vi "8_2.vi"() -> ()   [LabVIEW 2021, in "2023.lvlib"]
uses:
  2023.lvlib
panel:
  out "x*y":i64
  out "product":i64
  out "lines":string[](array[string])
  in  "Demo / Real Input":bool
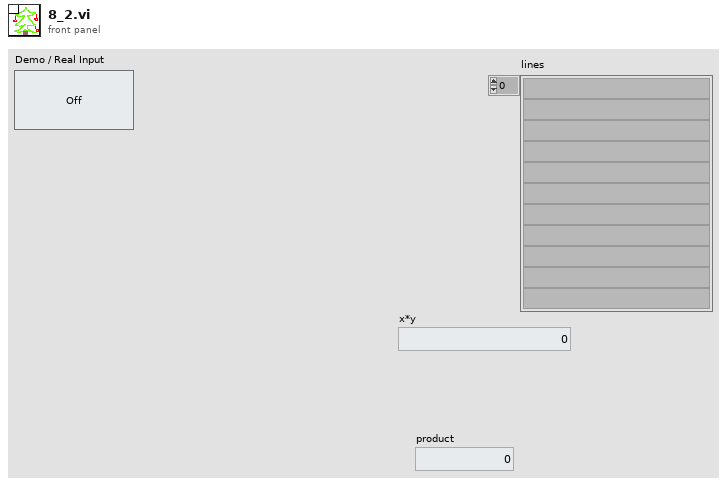
[diagram p1: front panel]
types:
  T1 = map{string, cluster{"LEFT":string, "RIGHT":string}}
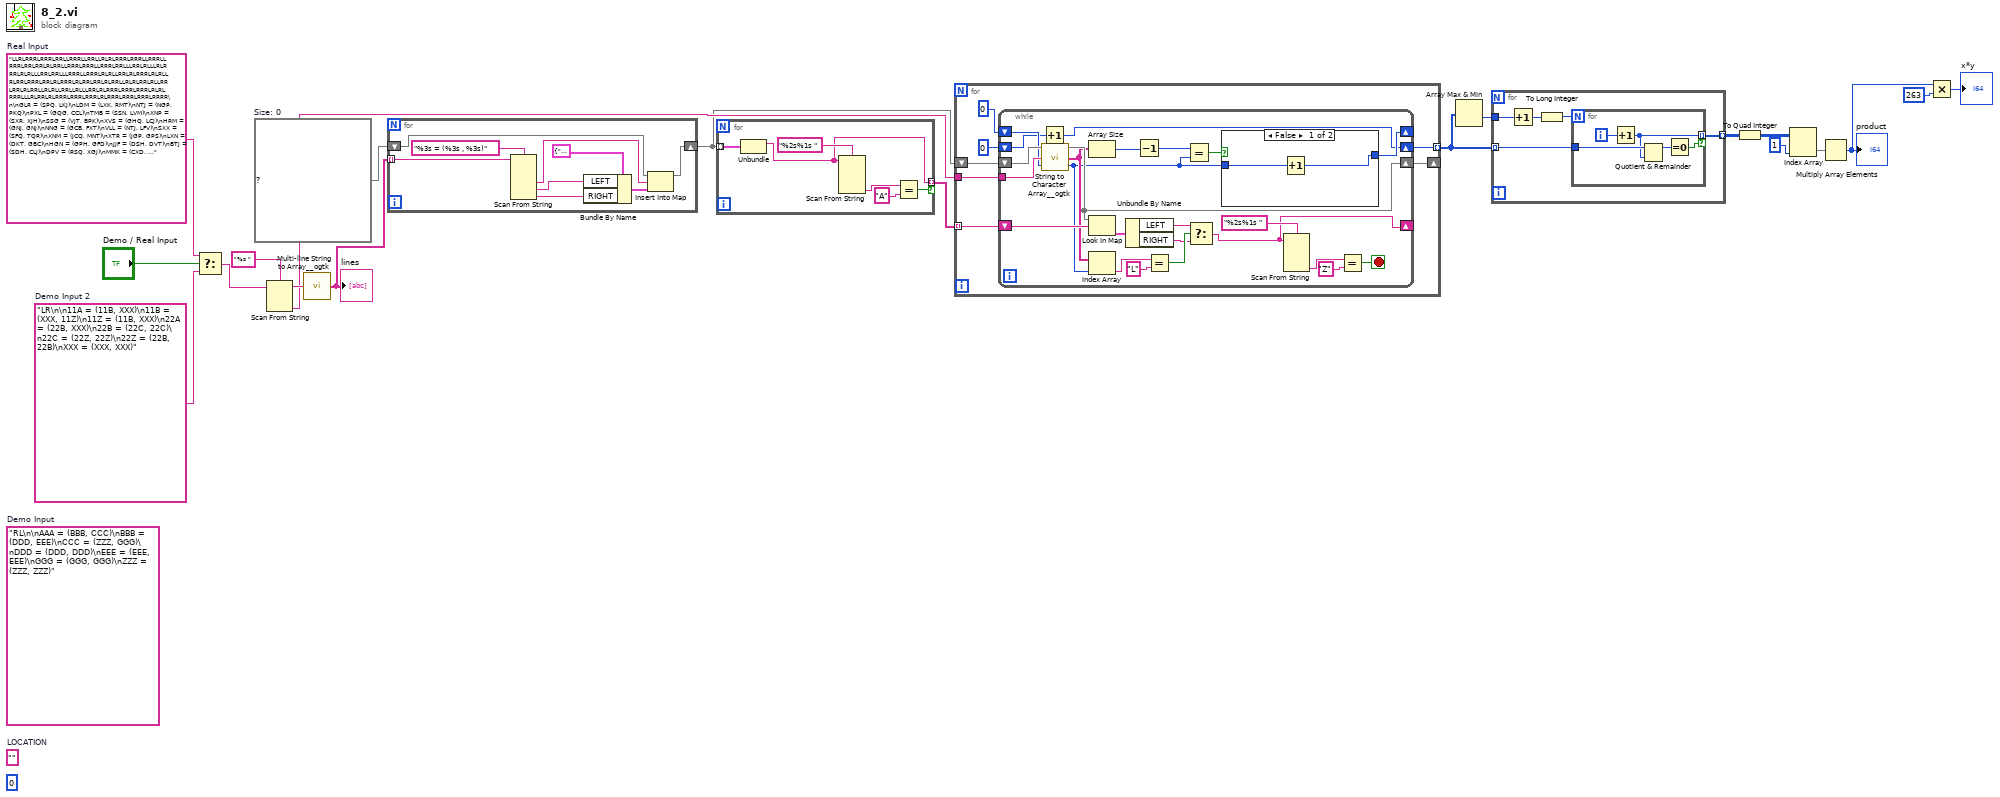
[diagram p0: block diagram]
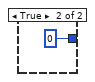
[diagram p2: hidden frame]
diagram:
  w13 = "LR\n\n11A = (11B, XXX)\n11B = (XXX, 11Z)\n11Z = (11B, XXX)\n22A = (22B, XXX)\n22B = (22C, 22C)\n22C = (22Z, 22Z)\n22Z = (22B, 22B)\nXXX = (XXX, XXX)"  # Demo Input 2
  (unwired) 0
  (unwired) ""  # LOCATION
  w14 = T1 {}  # Size: 0
  w20 = "LLRLRRRLRRRLRRLLRRRLLRRLLRLRLRRRLRRRLLRRRLLRRRLRRLRRLRLRRLLRRRLRRRLLRRRLRRLLLRRLRLLLRLRRRLRLRLLLRRLRRLLLRRRLLRRRLRLRLLRRLRLRRRLRLRLLRLRRLRRRLRRLRLRRRLRLRRLRRLRLRRLLRLRLRRLRLLRRLRRLRLRRLLRLRLLRRLLRLLLRRLRLRRRLRRRLRRRLRLRLRRRLLLRLRRLRLRRRLRRRLRRRLRLRRRLRRRLRRRLRRRR\n\nGLR = (SPQ, LKJ)\nLDM = (LXK, RMT)\nNTJ = (NGP, PKQ)\nPXL = (GQG, CCL)\nTMB = (SSN, LVM)\nXNP = (SXR, XJH)\nSSG = (VJT, BPK)\nXVS = (GHQ, LCJ)\nHRM = (GNJ, GNJ)\nNNG = (GCB, FXT)\nVLL = (NTJ, LFV)\nSXX = (SFQ, TQR)\nXNM = (JCQ, MNT)\nXTR = (JGP, GPS)\nLXN = (DKT, GBC)\nHGN = (GPH, GFD)\nJJF = (DSH, DVT)\nBTJ = (SDH, CLJ)\nDPV = (RSQ, XGJ)\nMMK = (CXD, KNV)\nFXT = (LDV, VBP)\nHDL = (RVD, JQG)\nGPX = (PFH, XBR)\nFMJ = (LJF, KPC)\nCRX = (XXN, XNQ)\nTQN = (JJF, SBZ)\nFGB = (JHR, QGC)\nHFQ = (PJS, FPN)\nBKS = (GCK, TRC)\nVPS = (BRP, BSL)\nJMV = (QQM, JVV)\nLMF = (DQJ, RQP)\nTDT = (KVD, KNT)\nPFP = (SMV, NXN)\nDKT = (NCT, MPG)\nNGP = (LMP, LBG)\nBPD = (HRM, HRM)\nCFK = (HDM, JSV)\nCLB = (PXL, CVB)\nGHG = (XVM, BGM)\nGCB = (LDV, VBP)\nNSH = (SHX, JTQ)\nGGR = (STX, HHQ)\nVTX = (XSM, TNV)\nJGB = (QTG, TBL)\nRDJ = (QQQ, NGC)\nKVL = (MBG, CDD)\nLVM = (KLR, KVT)\nFRV = (XRD, CGJ)\nVMJ = (DDG, GQC)\nFDA = (BKF, MQC)\nDSC = (QRC, FMJ)\nCRQ = (GKT, RMR)\nQLC = (HHT, HLQ)\nFSN = (LHJ, XTT)\nRDP = (CNJ, SQD)\nXRJ = (MCV, MVT)\nKJD = (JRX, JCM)\nPXJ = (JGH, CMB)\nFCQ = (XKQ, MFB)\nFXK = (MSB, TVD)\nJNF = (TQR, SFQ)\nCJJ = (PXJ, QQJ)\nKNV = (FTH, RFL)\nHFH = (CBP, DPN)\nLHT = (PGK, DLD)\nGLC = (DTJ, BDD)\nPNH = (SSG, QGT)\nPJS = (FHQ, GBD)\nNQJ = (XSD, KKD)\nXVL = (PGN, KSB)\nFMM = (CKQ, FVF)\nNFL = (BPV, HGF)\nPJR = (SNT, HBM)\nJQG = (XNM, QKN)\nNGQ = (NMV, NBS)\nCQV = (MXC, DQR)\nHQJ = (GGR, VCX)\nTTQ = (HLJ, MVF)\nHNR = (JGP, GPS)\nLRK = (NFL, LGC)\nGML = (TSF, HFT)\nNLV = (JQS, HHF)\nVGR = (VQT, DRX)\nTQR = (SXH, QJP)\nHPC = (PTF, RRH)\nKCN = (PQP, VBQ)\nHTF = (VGR, TTS)\nQKH = (DCP, KNL)\nHHH = (PJR, RSP)\nQMD = (FNP, CCG)\nLGV = (LTB, JST)\nKQX = (SPF, MLD)\nPJX = (MMP, RHG)\nQRD = (GDL, BBQ)\nCCG = (PVB, GBB)\nCPG = (KSD, BXG)\nPFV = (PMX, RHS)\nVCC = (RPQ, RDD)\nCVF = (XSM, TNV)\nQQX = (HGN, GDF)\nQVJ = (HXJ, GTV)\nPSD = (CQD, QFD)\nDLP = (QQX, SQR)\nHBM = (MCR, XVP)\nSFS = (BTS, TSC)\nNKN = (GBQ, RSF)\nVQT = (BTJ, FGM)\nXBH = (RMT, LXK)\nSRM = (PGK, DLD)\nFKQ = (SRV, PCC)\nLSX = (XVS, HMG)\nCLL = (NXN, SMV)\nGDD = (NLD, TGL)\nRVD = (XNM, QKN)\nRHG = (BJM, NBR)\nKFX = (FMJ, QRC)\nFGM = (CLJ, SDH)\nXJJ = (CVF, VTX)\nNHL = (XBJ, HLF)\nVMS = (VVQ, PPC)\nJCQ = (CFP, FGB)\nPSP = (VTH, HDC)\nLRQ = (GDG, VBL)\nPKL = (SSG, QGT)\nLHJ = (HML, JMG)\nBDX = (FMK, XDS)\nDPX = (BBF, SBK)\nGFD = (XVV, CHS)\nPSR = (FPP, DSL)\nHQB = (MRL, DHG)\nGKD = (SSP, JSP)\nTKL = (KBV, GTH)\nHMF = (HHT, HLQ)\nDGS = (VDJ, TJN)\nMRQ = (QVM, KJC)\nXSD = (TGJ, BDS)\nGDG = (RGS, HFH)\nJSV = (MFD, HXP)\nHMG = (LCJ, GHQ)\nBPV = (MRQ, XRL)\nSSP = (KQM, NSX)\nSDH = (QQR, RGR)\nJTX = (NHL, TST)\nNBR = (BXP, LSX)\nPCN = (JGR, PQQ)\nQCR = (RQV, FRV)\nNPH = (HHH, MXN)\nCBS = (PMX, RHS)\nJNR = (HKQ, XHG)\nGKT = (HRC, KHL)\nCDX = (NXJ, FVH)\nMXN = (RSP, PJR)\nZZZ = (VBQ, PQP)\nMSD = (VVQ, PPC)\nSMV = (VKQ, JNR)\nKKJ = (PGN, KSB)\nRJC = (CNM, LGB)\nQFB = (QQS, TMC)\nSTX = (KMP, KMP)\nQQR = (XTR, HNR)\nBPA = (DSH, DVT)\nGDT = (XVD, DNS)\nKXM = (CNJ, SQD)\nCHL = (LBP, PJX)\nXQX = (CMN, QXH)\nGQG = (BKS, VPQ)\nHRC = (VCR, NPH)\nLSL = (FMM, JTP)\nDDQ = (XPS, DMJ)\nDMF = (DHG, MRL)\nHBP = (KQX, CDN)\nDSR = (QMD, PBN)\nSJD = (VGP, KSG)\nPQQ = (KKJ, XVL)\nXQG = (LQK, GXD)\nQGT = (VJT, BPK)\nKDF = (LHG, LHG)\nVQV = (CGG, HVC)\nVJT = (XKS, CLB)\nTBL = (JSG, XDL)\nTCC = (DVX, KMN)\nSHP = (QRD, HDF)\nCRD = (FXQ, TVC)\nTQP = (FQN, BNF)\nJVV = (VMJ, VJS)\nLKJ = (KNP, GHG)\nDTR = (KHX, GQK)\nFXR = (GDT, GLK)\nDLD = (LBV, TMB)\nPNV = (BMP, LLQ)\nTMC = (FQV, PPS)\nVCR = (MXN, HHH)\nQSR = (DCP, KNL)\nNVT = (GNR, FKQ)\nJHM = (NLH, KQR)\nLBG = (TCC, RRN)\nPBK = (XBM, RJL)\nCGD = (PQQ, JGR)\nLHG = (JJF, JJF)\nFMD = (LGC, NFL)\nXJH = (LMF, SMX)\nCNM = (VBN, LGV)\nPPS = (NLV, VJR)\nGNN = (VQV, PLF)\nDXD = (SXR, XJH)\nVPQ = (GCK, TRC)\nKSB = (FSX, RJC)\nCQH = (VCC, RGM)\nDQV = (CBM, JGF)\nJPG = (MMQ, DLP)\nPNT = (BMB, TCS)\nMVF = (MNN, DFP)\nXVD = (PVR, CFK)\nDQR = (MBF, FCQ)\nHLF = (GGF, JPG)\nCFJ = (DPX, MHN)\nMDF = (LRK, FMD)\nGQT = (JTL, QRJ)\nKKR = (CJG, LST)\nBKF = (HDL, GCP)\nHGF = (XRL, MRQ)\nMCR = (CRR, BLQ)\nGVD = (BKF, MQC)\nJSG = (QRG, BCL)\nRQK = (XNQ, XXN)\nNXF = (NGQ, JSQ)\nRDD = (XNR, LVG)\nQJP = (GRS, QKX)\nRCL = (MDC, FJM)\nLXK = (CVG, BDX)\nKNP = (XVM, BGM)\nMPG = (NBF, KRK)\nCCL = (VPQ, BKS)\nSSN = (KVT, KLR)\nQRK = (FKH, VFD)\nQQS = (PPS, FQV)\nCHS = (NJX, QRK)\nPVL = (JRX, JCM)\nKNF = (HXJ, GTV)\nFKH = (CSV, JHP)\nXDK = (XQX, VHT)\nJKR = (MDR, NKN)\nDMJ = (KQL, BRM)\nKBV = (DSC, KFX)\nBRM = (BPD, NCB)\nSNT = (MCR, XVP)\nCFP = (JHR, QGC)\nTJF = (SRH, SLM)\nLMP = (TCC, RRN)\nCDM = (CVF, VTX)\nGQK = (NVT, TSJ)\nRGM = (RPQ, RDD)\nBLF = (HDC, VTH)\nPGS = (JRH, DPV)\nLCX = (QCD, XQG)\nGKM = (GLB, CJJ)\nGFB = (QCF, VNT)\nVQM = (PJP, PJP)\nHKH = (SHP, GCC)\nSTG = (GNN, VPZ)\nSBF = (KCN, ZZZ)\nKRK = (TTQ, CGX)\nVRF = (GLC, NXP)\nJFP = (QHG, RDJ)\nHDC = (SML, HPC)\nTPB = (GNJ, SBF)\nDDG = (DLT, KBM)\nQTM = (KDL, DVR)\nSJG = (NXJ, FVH)\nRTT = (QCF, VNT)\nGTV = (DMX, GFN)\nSBK = (DJD, VFS)\nXVP = (BLQ, CRR)\nLXP = (TQP, BBX)\nCMB = (PVL, KJD)\nVHT = (QXH, CMN)\nSMR = (LST, CJG)\nBXG = (XBF, XFD)\nGXD = (NPV, HBP)\nBVA = (SMR, KKR)\nXRD = (SQN, MVX)\nCNJ = (BMK, RPT)\nQFR = (LRK, FMD)\nFPP = (NCR, VPS)\nNQN = (LBP, PJX)\nPLF = (CGG, HVC)\nTPK = (VQM, VQM)\nMKK = (MTJ, PSD)\nPFB = (MXP, LGF)\nVDJ = (LSL, QVX)\nFVH = (JXQ, PBK)\nHDM = (HXP, MFD)\nVJS = (DDG, GQC)\nPHC = (KDF, TCB)\nVFD = (CSV, JHP)\nRRH = (GDD, XDM)\nMRL = (GML, DLB)\nCDD = (JDK, KJQ)\nXPS = (KQL, BRM)\nNXH = (JMV, PVK)\nNJX = (FKH, VFD)\nFQL = (DSL, FPP)\nLST = (QDF, JDR)\nPQP = (LHT, SRM)\nLPS = (PTK, PHC)\nCVT = (CXD, KNV)\nQTG = (XDL, JSG)\nFXQ = (FGC, QBT)\nTRK = (SSQ, LPX)\nPTK = (KDF, KDF)\nBXP = (HMG, XVS)\nGCK = (QVJ, KNF)\nMSB = (QKR, NQJ)\nSVN = (DPV, JRH)\nCQD = (PST, DQV)\nQBQ = (TNG, PNT)\nHJZ = (MQC, BKF)\nHPT = (GDG, VBL)\nTJN = (QVX, LSL)\nNDA = (VQV, PLF)\nJHP = (XRJ, VKF)\nQTP = (XTT, LHJ)\nJTL = (GVD, GVD)\nDDV = (NDJ, NVK)\nSCF = (VCC, RGM)\nRGL = (NSH, TMK)\nKSD = (XBF, XFD)\nRJL = (TPK, BVS)\nQKX = (NPC, PPG)\nXMR = (TBL, QTG)\nCVG = (FMK, XDS)\nSKS = (SVQ, THL)\nCCM = (MXP, LGF)\nTNG = (TCS, BMB)\nXXN = (GLR, QQK)\nNVK = (VRF, PMC)\nRRN = (DVX, KMN)\nNPC = (LJH, LJH)\nJJL = (XBH, LDM)\nLDV = (FXK, DMP)\nKMP = (JTL, JTL)\nQNQ = (RMR, GKT)\nJXQ = (XBM, RJL)\nCBP = (NQN, CHL)\nPPG = (LJH, XTG)\nLQK = (HBP, NPV)\nXTT = (HML, JMG)\nSVQ = (PKL, PNH)\nDSL = (NCR, VPS)\nLTB = (FKX, DTR)\nNLH = (GFB, RTT)\nQFD = (PST, DQV)\nRHS = (SNV, HPJ)\nJPT = (GCS, VGX)\nVTH = (HPC, SML)\nJRF = (LNR, HSF)\nBPK = (CLB, XKS)\nLHH = (RDP, KXM)\nTKP = (DQF, CXL)\nXVV = (NJX, QRK)\nGBD = (MBC, QBQ)\nPBP = (DDV, THT)\nTNF = (KNT, KVD)\nRFL = (VMX, DBF)\nMBC = (TNG, PNT)\nMCV = (VDS, PBP)\nGNR = (PCC, SRV)\nDHG = (GML, DLB)\nTCV = (LDF, TKL)\nXDS = (PSR, FQL)\nVMR = (TST, NHL)\nXVM = (RGK, QFB)\nLJN = (MXC, DQR)\nVBL = (HFH, RGS)\nLCG = (PFV, CBS)\nSXR = (LMF, SMX)\nTGL = (VMR, JTX)\nBDS = (QKH, QSR)\nRGS = (CBP, DPN)\nRFZ = (KKR, SMR)\nJTQ = (DSR, BQJ)\nBQJ = (QMD, PBN)\nVVQ = (DGS, GSN)\nCGG = (NNL, LCR)\nCVH = (LPX, SSQ)\nNGC = (GKM, TTN)\nXNR = (XNP, DXD)\nFBN = (DQF, CXL)\nMBG = (KJQ, JDK)\nJSQ = (NMV, NBS)\nLRF = (VJM, MQQ)\nGBC = (NCT, MPG)\nNXP = (BDD, DTJ)\nLGC = (BPV, HGF)\nHDF = (BBQ, GDL)\nRSF = (JPT, SCP)\nLDF = (KBV, GTH)\nQQJ = (CMB, JGH)\nSHX = (DSR, BQJ)\nRSP = (SNT, HBM)\nGPH = (CHS, XVV)\nDQJ = (QNQ, CRQ)\nMMQ = (SQR, QQX)\nFVF = (PCN, CGD)\nBBF = (VFS, DJD)\nQBT = (HFQ, PGM)\nRPQ = (XNR, LVG)\nCJG = (QDF, JDR)\nSBR = (MSD, VMS)\nSXH = (GRS, QKX)\nMFB = (JTF, QTM)\nDBL = (XBR, PFH)\nTGJ = (QSR, QKH)\nCXL = (KMK, RVR)\nPGM = (FPN, PJS)\nNMR = (HXM, TJF)\nQGC = (STV, NJT)\nVMX = (GTG, QCR)\nDSH = (CRX, RQK)\nPST = (CBM, JGF)\nJVR = (PVK, JMV)\nGRS = (NPC, NPC)\nRBT = (MHN, DPX)\nXBF = (XQL, BVB)\nDJD = (CFF, JJL)\nGLB = (PXJ, QQJ)\nMQC = (HDL, GCP)\nSHC = (BKK, STG)\nJGH = (PVL, KJD)\nXHG = (VVS, HTD)\nSPF = (XMR, JGB)\nGHV = (BLF, PSP)\nVGN = (KSG, VGP)\nFQV = (NLV, VJR)\nHHR = (LJN, CQV)\nGFN = (FHL, SHC)\nKJQ = (NXH, JVR)\nCFF = (XBH, LDM)\nSFQ = (SXH, QJP)\nXBR = (CQH, SCF)\nXND = (DMJ, XPS)\nLDQ = (BXG, KSD)\nCMN = (PFP, CLL)\nGCC = (HDF, QRD)\nHPJ = (PMP, FRM)\nBSS = (MKK, TVJ)\nVTC = (DKR, MXS)\nVCX = (STX, HHQ)\nRQV = (XRD, CGJ)\nPGK = (TMB, LBV)\nHTD = (LRF, KXL)\nPVR = (JSV, HDM)\nBBQ = (XKC, HHR)\nPKQ = (LBG, LMP)\nNCN = (GGR, VCX)\nPBN = (FNP, CCG)\nSQD = (BMK, RPT)\nQKR = (KKD, XSD)\nDTJ = (DGX, LPB)\nTSJ = (GNR, FKQ)\nTVC = (FGC, QBT)\nNCC = (RGL, KGL)\nDVT = (CRX, RQK)\nTHL = (PKL, PNH)\nQQM = (VMJ, VJS)\nDKR = (NCN, HQJ)\nMKF = (VLR, LQS)\nVFS = (CFF, JJL)\nGDF = (GFD, GPH)\nDQF = (RVR, KMK)\nNSX = (KLV, CLQ)\nJGF = (TCV, QDH)\nXKS = (PXL, CVB)\nRSQ = (HQB, DMF)\nDXX = (LFV, NTJ)\nVKF = (MCV, MVT)\nBDD = (DGX, LPB)\nDNS = (PVR, CFK)\nSRV = (RQC, JHM)\nXDL = (QRG, BCL)\nNCT = (KRK, NBF)\nXQK = (THL, SVQ)\nDLB = (HFT, TSF)\nDVX = (CJF, NSJ)\nNCR = (BSL, BRP)\nCSV = (XRJ, VKF)\nKLS = (TTS, VGR)\nJCB = (BLM, TQL)\nMXP = (NNG, XXS)\nFNP = (PVB, GBB)\nXGS = (GLK, GDT)\nVBQ = (SRM, LHT)\nGHQ = (SJG, CDX)\nLQS = (JKR, XDX)\nMXS = (HQJ, NCN)\nMNN = (TKP, FBN)\nDVR = (CVH, TRK)\nVKQ = (HKQ, XHG)\nKHX = (TSJ, NVT)\nBMK = (SKB, JCB)\nFGC = (HFQ, PGM)\nTVD = (QKR, NQJ)\nBNF = (CFJ, RBT)\nNXN = (VKQ, JNR)\nVJM = (CCS, KVL)\nXRL = (QVM, KJC)\nSRH = (XJJ, CDM)\nFDF = (JNF, SXX)\nXKM = (FDV, VTC)\nBLQ = (CDT, CRD)\nVMF = (QLC, HMF)\nJGP = (LPS, JNC)\nBVB = (HPT, LRQ)\nLNR = (QFR, MDF)\nVJR = (HHF, JQS)\nFHQ = (MBC, QBQ)\nSLM = (XJJ, CDM)\nHVC = (LCR, NNL)\nKNT = (XKM, VDF)\nKGL = (NSH, TMK)\nKNL = (GKD, SBM)\nCJF = (VGN, SJD)\nHXJ = (DMX, GFN)\nRGR = (XTR, HNR)\nPMP = (XDK, HLS)\nTKB = (BLF, PSP)\nVBJ = (RGL, KGL)\nLCJ = (CDX, SJG)\nJCM = (HKH, KDS)\nCXD = (FTH, RFL)\nTSF = (CXS, NXF)\nBSL = (CCM, PFB)\nQRC = (KPC, LJF)\nMLD = (JGB, XMR)\nCRR = (CRD, CDT)\nGNJ = (KCN, KCN)\nQRJ = (GVD, HJZ)\nCDN = (SPF, MLD)\nHLS = (VHT, XQX)\nHML = (SBR, FMH)\nRPT = (JCB, SKB)\nSBM = (SSP, JSP)\nVBN = (LTB, JST)\nNBS = (FDF, MSG)\nMDR = (GBQ, RSF)\nXDM = (TGL, NLD)\nSKB = (TQL, BLM)\nNNL = (LXP, QTD)\nKQM = (KLV, CLQ)\nVLR = (JKR, XDX)\nRSG = (LDQ, CPG)\nLJH = (NMR, NMR)\nRGK = (QQS, TMC)\nSQN = (VVL, JFP)\nDFP = (TKP, FBN)\nSCP = (VGX, GCS)\nVBP = (DMP, FXK)\nNMV = (MSG, FDF)\nQCF = (DXX, VLL)\nHHT = (MKF, GBN)\nSBZ = (DVT, DSH)\nSNV = (PMP, FRM)\nGQC = (KBM, DLT)\nMQQ = (KVL, CCS)\nVGP = (LXN, MVD)\nGBN = (VLR, LQS)\nMVX = (JFP, VVL)\nDRX = (BTJ, FGM)\nJRH = (XGJ, RSQ)\nRVR = (TDT, TNF)\nPVK = (QQM, JVV)\nJQS = (XGS, FXR)\nBCL = (RSG, QSL)\nGBB = (MMK, CVT)\nSSQ = (XND, DDQ)\nPCC = (JHM, RQC)\nCCS = (CDD, MBG)\nMMP = (NBR, BJM)\nMTJ = (QFD, CQD)\nPVB = (CVT, MMK)\nKLR = (TND, VMF)\nFKX = (KHX, GQK)\nFDV = (DKR, MXS)\nTCB = (LHG, TQN)\nJDK = (NXH, JVR)\nGBQ = (SCP, JPT)\nTTN = (GLB, CJJ)\nJTF = (DVR, KDL)\nQQQ = (TTN, GKM)\nDXP = (LHH, CSF)\nMFD = (BSS, PQJ)\nPGN = (RJC, FSX)\nMBF = (XKQ, MFB)\nXXS = (FXT, GCB)\nVGX = (VBJ, NCC)\nFPJ = (PJP, RFZ)\nXTG = (NMR, PQZ)\nJGR = (XVL, KKJ)\nMSG = (JNF, SXX)\nCKQ = (PCN, CGD)\nQSL = (LDQ, CPG)\nXQL = (HPT, LRQ)\nKVT = (TND, VMF)\nBBX = (BNF, FQN)\nCLJ = (QQR, RGR)\nGSN = (VDJ, TJN)\nDLT = (SXP, SFS)\nXFD = (BVB, XQL)\nFHL = (BKK, BKK)\nFSX = (LGB, CNM)\nSPQ = (KNP, GHG)\nNXJ = (JXQ, PBK)\nNPV = (CDN, KQX)\nDPN = (CHL, NQN)\nRMR = (HRC, KHL)\nLPF = (XQG, QCD)\nTHT = (NDJ, NVK)\nJNC = (PTK, PHC)\nLGF = (XXS, NNG)\nCVB = (CCL, GQG)\nVVL = (RDJ, QHG)\nLCR = (LXP, QTD)\nPQJ = (TVJ, MKK)\nVDF = (FDV, VTC)\nGTG = (FRV, RQV)\nFRM = (XDK, HLS)\nLPB = (SPV, PNV)\nNBF = (TTQ, CGX)\nXKQ = (QTM, JTF)\nBRP = (PFB, CCM)\nKVD = (XKM, VDF)\nXBJ = (GGF, JPG)\nKDS = (GCC, SHP)\nTVJ = (PSD, MTJ)\nXSM = (NLJ, JRF)\nBTS = (SKS, XQK)\nVVS = (LRF, KXL)\nSPV = (BMP, LLQ)\nKQL = (BPD, NCB)\nCGX = (MVF, HLJ)\nXBM = (TPK, TPK)\nTMK = (JTQ, SHX)\nVNT = (DXX, VLL)\nCBM = (QDH, TCV)\nTQL = (QTP, FSN)\nHKQ = (VVS, HTD)\nRQC = (KQR, NLH)\nFMH = (VMS, MSD)\nNCB = (HRM, TPB)\nBKK = (GNN, GNN)\nQRG = (QSL, RSG)\nJSP = (NSX, KQM)\nRQP = (CRQ, QNQ)\nJHR = (NJT, STV)\nMXC = (MBF, FCQ)\nLBV = (LVM, SSN)\nKLV = (KFG, RCL)\nFJM = (TXK, LCG)\nQVX = (FMM, JTP)\nLJF = (KLS, HTF)\nQXH = (PFP, CLL)\nKQR = (GFB, RTT)\nMHN = (SBK, BBF)\nGTH = (KFX, DSC)\nGCP = (RVD, JQG)\nCXS = (NGQ, JSQ)\nBJM = (BXP, LSX)\nLLQ = (NRD, FSK)\nCSF = (RDP, KXM)\nTXK = (CBS, PFV)\nSXP = (TSC, BTS)\nPQZ = (TJF, HXM)\nKBM = (SXP, SFS)\nHHF = (FXR, XGS)\nTNV = (NLJ, JRF)\nJST = (DTR, FKX)\nXKC = (LJN, CQV)\nTCS = (SVN, PGS)\nPPC = (DGS, GSN)\nLGB = (LGV, VBN)\nMVT = (VDS, PBP)\nTST = (XBJ, HLF)\nQVM = (GPX, DBL)\nNSJ = (SJD, VGN)\nPFH = (SCF, CQH)\nJTP = (FVF, CKQ)\nQDF = (GHV, TKB)\nTTS = (DRX, VQT)\nCDT = (FXQ, TVC)\nDCP = (SBM, GKD)\nVPZ = (PLF, VQV)\nNLD = (JTX, VMR)\nHFT = (CXS, NXF)\nGCS = (VBJ, NCC)\nHHQ = (KMP, GQT)\nRMT = (BDX, CVG)\nTRC = (QVJ, KNF)\nLPX = (DDQ, XND)\nSQR = (HGN, GDF)\nKFG = (MDC, FJM)\nBGM = (RGK, QFB)\nKKD = (TGJ, BDS)\nLFV = (PKQ, NGP)\nGPS = (LPS, JNC)\nCGJ = (MVX, SQN)\nDGX = (SPV, PNV)\nKMK = (TDT, TNF)\nBVS = (VQM, FPJ)\nMDC = (TXK, LCG)\nKMN = (CJF, NSJ)\nQHG = (QQQ, NGC)\nKXL = (VJM, MQQ)\nBMB = (SVN, PGS)\nNLJ = (LNR, HSF)\nTSC = (XQK, SKS)\nJRX = (KDS, HKH)\nTND = (QLC, HMF)\nQCD = (LQK, GXD)\nNRD = (LCX, LPF)\nHXP = (PQJ, BSS)\nHLJ = (MNN, DFP)\nMNT = (CFP, FGB)\nKSG = (MVD, LXN)\nFPN = (FHQ, GBD)\nHXM = (SRH, SLM)\nCLQ = (KFG, RCL)\nXGJ = (DMF, HQB)\nFSK = (LPF, LCX)\nGDL = (HHR, XKC)\nPTF = (XDM, GDD)\nAAA = (PQP, VBQ)\nXDX = (MDR, NKN)\nSMX = (RQP, DQJ)\nLBP = (RHG, MMP)\nFQN = (RBT, CFJ)\nKDL = (CVH, TRK)\nQCA = (HXM, TJF)\nMVD = (GBC, DKT)\nFMK = (FQL, PSR)\nPMX = (SNV, HPJ)\nGLK = (XVD, DNS)\nNJT = (DXP, XHQ)\nSML = (RRH, PTF)\nBMP = (NRD, FSK)\nQKN = (MNT, JCQ)\nQQK = (SPQ, LKJ)\nJDR = (GHV, TKB)\nDMX = (FHL, FHL)\nPMC = (NXP, GLC)\nHSF = (QFR, MDF)\nNDJ = (PMC, VRF)\nJMG = (SBR, FMH)\nKHL = (NPH, VCR)\nQTD = (BBX, TQP)\nXHQ = (LHH, CSF)\nGGF = (DLP, MMQ)\nQDH = (TKL, LDF)\nDMP = (MSB, TVD)\nBLM = (QTP, FSN)\nDBF = (QCR, GTG)\nXNQ = (QQK, GLR)\nHLQ = (MKF, GBN)\nVDS = (DDV, THT)\nLVG = (XNP, DXD)\nSTV = (XHQ, DXP)\nKPC = (HTF, KLS)\nFTH = (VMX, DBF)\nKJC = (DBL, GPX)\nPJP = (SMR, KKR)"  # Real Input
  (unwired) "RL\n\nAAA = (BBB, CCC)\nBBB = (DDD, EEE)\nCCC = (ZZZ, GGG)\nDDD = (DDD, DDD)\nEEE = (EEE, EEE)\nGGG = (GGG, GGG)\nZZZ = (ZZZ, ZZZ)"  # Demo Input
  n1 = Select(t=w20, s="Demo / Real Input", f=w13) -> (s? t:f=w18:string)
  n2 = Scan From String(format string="%s ", input string=w18) -> (remaining string=w16:string, output 1=w11:string)  [unwired: 3 in, 2 out]
  n3 = call <userlib>:"Multi-line String to Array__ogtk.vi"("string"=w16) -> ("lines"=w15:string[])
  "lines" <- w15
  n4 = for {
    tunnel: w15 -> [w29] mode=indexing
    shift-right: [w21] -> w10
    shift-left: w14 -> [w27]
    n5 = Scan From String(format string="%3s = (%3s , %3s)", input string=w29) -> (output 1=w26:string, output 2=w24:string, output 3=w23:string)  [unwired: 5 in, 3 out]
    n6 = Bundle By Name(cluster=cluster{"LEFT":string, "RIGHT":string} {"LEFT"="", "RIGHT"=""}, "LEFT"=w24, "RIGHT"=w23) -> (w22:cluster{"LEFT":string, "RIGHT":string})
    n7 = Insert Into Map(map in=w27, key=w26, value=w22) -> (map out=w21:T1)  [unwired: 2 out]
  }
  n8 = for {
    tunnel: w10 -> [w35] mode=indexing
    tunnel: [w30] -> w12 mode=indexing if=w32
    n9 = Unbundle(w35) -> (w30:string)  [unwired: 1 out]
    n10 = Scan From String(format string="%2s%1s ", input string=w30) -> (output 2=w31:string)  [unwired: 5 in, 3 out]
    n11 = Equal?(x=w31, y="A") -> (x = y?=w32:bool)
  }
  n12 = for {
    tunnel: w12 -> [w41] mode=indexing
    tunnel: w11 -> [w40]
    shift-right: [w37] -> _
    shift-left: w10 -> [w39]
    tunnel: [w36] -> w2 mode=indexing
    n13 = while {
      shift-right: [w61] -> w37
      shift-left: w39 -> [w61]
      tunnel: w40 -> [w64]
      shift-right: [w63] -> _
      shift-left: 0 -> [w56]
      shift-right: [w44] -> _
      shift-left: w41 -> [w60]
      shift-right: [w54] -> w36
      shift-left: i64 0 -> [w55]
      stop <- w43 stop-if-true
      n14 = Increment(x=w55) -> (x+1=w54:i64)
      n15 = call <userlib>:"String to Character Array__ogtk.vi"("Input String"=w64) -> ("Character Array"=w57:string[])
      n16 = Array Size(array=w57) -> (size(s)=w59:i32)
      n17 = Look In Map(map=w61, key=w60) -> (value=w50:cluster{"LEFT":string, "RIGHT":string})  [unwired: 1 in, 1 out]
      n18 = Index Array(array=w57, index=w56) -> (element=w53:string)
      n19 = Unbundle By Name(w50) -> ("LEFT"=w49:string, "RIGHT"=w48:string)
      n20 = Decrement(x=w59) -> (x-1=w58:i32)
      n21 = Equal?(x=w53, y="L") -> (x = y?=w51:bool)
      n22 = Equal?(x=w58, y=w56) -> (x = y?=w62:bool)
      n23 = Select(t=w49, s=w51, f=w48) -> (s? t:f=w44:string)
      n24 = case shown="False" w62 {
        tunnel: w56 -> [w66 _]
        tunnel: [w65 0] -> w63
        frame False {
          n25 = Increment(x=w66) -> (x+1=w65:i32)
        }
        frame True {
        }
      }
      n26 = Scan From String(format string="%2s%1s ", input string=w44) -> (output 2=w47:string)  [unwired: 5 in, 3 out]
      n27 = Equal?(x=w47, y="Z") -> (x = y?=w43:bool)
    }
  }
  n28 = Array Max & Min(array=w2) -> (min value=w1:i64)  [unwired: 3 out]
  n29 = for {
    tunnel: w2 -> [w72] mode=indexing
    tunnel: [w71] -> w9 mode=indexing
    tunnel: w1 -> [w70]
    n30 = Increment(x=w70) -> (x+1=w69:i64)
    n31 = To Long Integer(number=w69) -> (32bit integer=w68:i32)
    n32 = for {
      N: w68 -> [_]
      tunnel: w72 -> [w77]
      tunnel: [w73] -> w71 mode=indexing if=w74
      i -> [w76]
      n33 = Increment(x=w76) -> (x+1=w73:i32)
      n34 = Quotient & Remainder(x=w77, y=w73) -> (x-y*floor(x/y)=w75:i64)  [unwired: 1 out]
      n35 = Equal To 0?(x=w75) -> (x = 0?=w74:bool)
    }
  }
  n36 = To Quad Integer(1:w9) -> (0:w6:i64[][])
  n37 = Index Array(array=w6, index (col)=1 ("disabled index (col)")) -> (element=w7:i64[])  [unwired: 1 in]
  n38 = Multiply Array Elements(1:w7) -> (0:w5:i64)
  "product" <- w5
  n39 = Multiply(x=w5, y=i64 263) -> (x*y=→"x*y":i64)
